vi "Plot Line (SubVI).vi"(8 "Polar Graph Attributes":T2, 9 "Draw Area Size":T1, 10 "Polar Array":cluster{"magnitude":dbl, "phase":dbl}[](array[cluster]), 11 "new picture in":picture) -> (3 "new picture out":picture)   [LabVIEW 2021]
uses:
  <vilib>/Utility/miscctls.llb/LVBoundsTypeDef.ctl
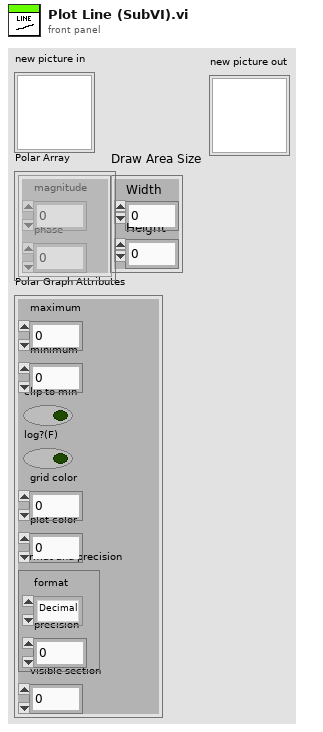
[diagram p1: front panel]
types:
  T1 = typedef "LVBoundsTypeDef.ctl" = cluster{"Width":u32, "Height":u32}
  T2 = cluster{"maximum":dbl, "minimum":dbl, "clip to min":bool, "log?(F)":bool, "grid color":u32, "plot color":u32, "format and precision":cluster{"format":enum8{"Decimal", "Scientific", "Engineering", "Binary", "Octal", "Hex"}, "precision":u8}, "visible section":u16}
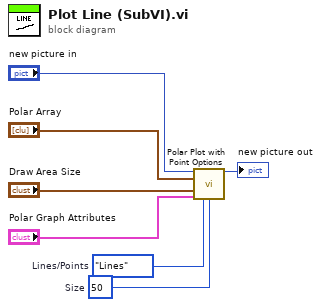
[diagram p0: block diagram]
diagram:
  w3 = u16 50  # Size
  w4 = enum16{"Lines", "Points"}."Lines"  # Lines/Points
  n1 = call <vilib>:"Polar Plot with Point Options.vi"("picture"="new picture in", "data array [mag, phase (deg)]"="Polar Array", "dimensions (w,h)"="Draw Area Size", "polar attributes"="Polar Graph Attributes", "Lines/Points"=w4, "Size"=w3) -> ("new picture"=→"new picture out":picture)  [unwired: 9 in]
